vi "testFlattenForceToXML.vi"() -> ()   [LabVIEW 2012, in "UnitsAndXML.lvlib"]
uses:
  <userlib>/Common/UnitsAndXML/UnitsAndXML.lvlib
  <userlib>/Common/UnitsAndXML/FlattenItemWithUnitToXML/FlattenForceToXML/ForceUnit.ctl
  <userlib>/Common/UnitsAndXML/FlattenItemWithUnitToXML/FlattenForceToXML/typeMethods/flattenForceToXML_Array.vi
  <userlib>/Common/UnitsAndXML/FlattenItemWithUnitToXML/FlattenForceToXML/typeMethods/flattenForceToXML_Scalar.vi
panel:
  out "error out":errorcluster
  in  "forceUnitInXML":T1
  out "xmlStringArray":string
  out "xmlStringScalar":string
  in  "force":dbl[unit][](array[numeric])=[66.72333, 133.44666, 200.16999, 266.89332]
  in  "force":dbl[unit]=66.72333
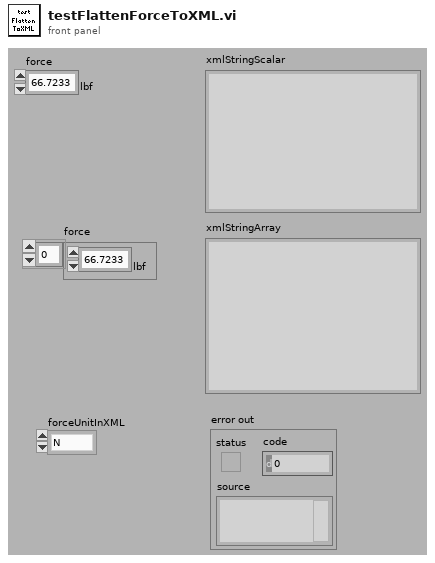
[diagram p1: front panel]
types:
  T1 = typedef "UnitsAndXML.lvlib/ForceUnit.ctl" = enum16{"N", "dyn", "lbf"}
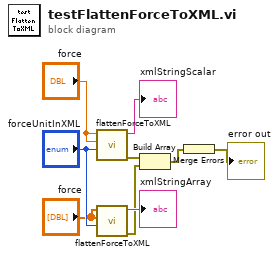
[diagram p0: block diagram]
diagram:
  n1 = call-poly <userlib>:"flattenForceToXML.vi"("forceUnitInXML"="forceUnitInXML", "forceAgain"="force", "force"="force") -> ("error out"=w6:errorcluster, "xmlString"=→"xmlStringScalar":string)  [unwired: 7 in]
  n2 = call-poly <userlib>:"flattenForceToXML.vi"("forceUnitInXML"="forceUnitInXML", "forceAgain"="force", "force"="force") -> ("error out"=w1:errorcluster, "xmlString"=→"xmlStringArray":string)  [unwired: 7 in]
  n3 = Build Array(w6, w1) -> (w7:errorcluster[])
  n4 = Merge Errors(w7) -> (→"error out":errorcluster)
